vi "Add New Or Old Parameter.vi"(8 "old port?":bool, 9 "refresh listbox":T4[](array[typedef]), 10 "channel parameter":T1={"name"="", "default value"=0.0, "unit"="", "Parameter"={"start index"=0, "size"=1, "encoding"=enum."BNR", "signed"=FALSE, "scale multiplier"=1.0, "scale offset"=0.0}}) -> (1 "refresh listbox out":T4[](array[typedef]))   [LabVIEW 2020, in "AIM ARINC 429 System Explorer.lvlib" / "Implementation.lvlib"]
uses:
  Implementation.lvlib
  Types/Refresh Listbox.ctl
  Types/Refresh Symbols.ctl
  Shared/VS Channel Definition for Parameter.ctl
  Shared/Parameter Definition.ctl
  <vilib>/NI/NI VeriStand Encoding and Decoding/Encoding.ctl
  Refresh Constants.vi
  <vilib>/NI/NI VeriStand Encoding and Decoding/Encoding and Decoding.lvlib
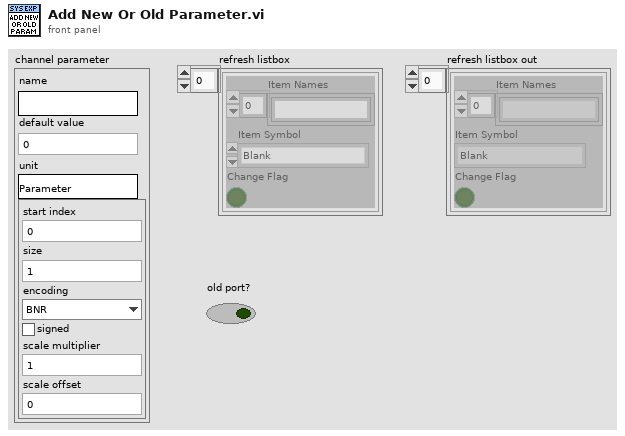
[diagram p1: front panel]
types:
  T1 = typedef "VS Channel Definition for Parameter.ctl" = cluster{"name":string, "default value":dbl, "unit":string, "Parameter":T2}
  T2 = typedef "Parameter Definition.ctl" = cluster{"start index":i32, "size":i32, "encoding":T3, "signed":bool, "scale multiplier":dbl, "scale offset":dbl}
  T3 = typedef "Encoding and Decoding.lvlib/Encoding.ctl" = enum16{"BNR", "BCD", "Discrete"}
  T4 = typedef "AIM ARINC 429 System Explorer.lvlib/Implementation.lvlib/Refresh Listbox.ctl" = cluster{"Item Names":string[], "Item Symbol":T5, "Change Flag":bool}
  T5 = typedef "AIM ARINC 429 System Explorer.lvlib/Implementation.lvlib/Refresh Symbols.ctl" = enum16{"Blank", "Port", "Incoming", "Outgoing", "Label", "Word", "Parameter", "ARINC-429", "Config Files", "Channel Spec", "Item"}
  T6 = typedef "AIM ARINC 429 System Explorer.lvlib/Implementation.lvlib/Parameter Strings.ctl" = cluster{"name":string, "default value":string, "unit":string, "start index":string, "size":string, "encoding":string, "signed":string, "scale multiplier":string, "scale offset":string}
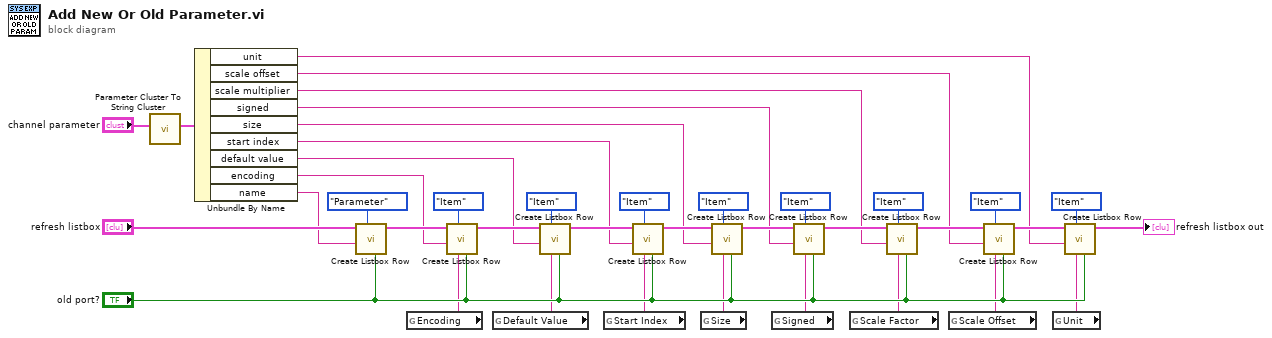
[diagram p0: block diagram]
diagram:
  n1 = call "Parameter Cluster To String Cluster.vi"("parameter"="channel parameter") -> ("parameter strings"=w18:T6)  [unwired: 10 in]
  n2 = Unbundle By Name(w18) -> ("unit"=w16:string, "scale offset"=w9:string, "scale multiplier"=w10:string, "signed"=w11:string, "size"=w12:string, "start index"=w13:string, "default value"=w14:string, "encoding"=w15:string, "name"=w17:string)
  n3 = call "Create Listbox Row.vi"("swap new and old (F)"="old port?", "refresh symbol (Blank)"=Refresh_Symbols."Parameter" ("Refresh Symbol (Blank)"), "new item"=w17, "refresh listbox"="refresh listbox") -> ("refresh listbox out"=w34:T4[])  [unwired: 7 in]
  n4 = global read "Refresh Constants.vi" "Encoding"() -> (w8:string)
  n5 = call "Create Listbox Row.vi"("swap new and old (F)"="old port?", "override name"=w8, "refresh symbol (Blank)"=Refresh_Symbols."Item" ("Refresh Symbol (Blank)"), "new item"=w15, "refresh listbox"=w34) -> ("refresh listbox out"=w32:T4[])  [unwired: 6 in]
  n6 = global read "Refresh Constants.vi" "Default Value"() -> (w7:string)
  n7 = call "Create Listbox Row.vi"("swap new and old (F)"="old port?", "override name"=w7, "refresh symbol (Blank)"=Refresh_Symbols."Item" ("Refresh Symbol (Blank)"), "new item"=w14, "refresh listbox"=w32) -> ("refresh listbox out"=w30:T4[])  [unwired: 6 in]
  n8 = global read "Refresh Constants.vi" "Start Index"() -> (w6:string)
  n9 = call "Create Listbox Row.vi"("swap new and old (F)"="old port?", "override name"=w6, "refresh symbol (Blank)"=Refresh_Symbols."Item" ("Refresh Symbol (Blank)"), "new item"=w13, "refresh listbox"=w30) -> ("refresh listbox out"=w28:T4[])  [unwired: 6 in]
  n10 = global read "Refresh Constants.vi" "Size"() -> (w5:string)
  n11 = call "Create Listbox Row.vi"("swap new and old (F)"="old port?", "override name"=w5, "refresh symbol (Blank)"=Refresh_Symbols."Item" ("Refresh Symbol (Blank)"), "new item"=w12, "refresh listbox"=w28) -> ("refresh listbox out"=w26:T4[])  [unwired: 6 in]
  n12 = global read "Refresh Constants.vi" "Signed"() -> (w4:string)
  n13 = call "Create Listbox Row.vi"("swap new and old (F)"="old port?", "override name"=w4, "refresh symbol (Blank)"=Refresh_Symbols."Item" ("Refresh Symbol (Blank)"), "new item"=w11, "refresh listbox"=w26) -> ("refresh listbox out"=w24:T4[])  [unwired: 6 in]
  n14 = global read "Refresh Constants.vi" "Scale Factor"() -> (w1:string)
  n15 = call "Create Listbox Row.vi"("swap new and old (F)"="old port?", "override name"=w1, "refresh symbol (Blank)"=Refresh_Symbols."Item" ("Refresh Symbol (Blank)"), "new item"=w10, "refresh listbox"=w24) -> ("refresh listbox out"=w22:T4[])  [unwired: 6 in]
  n16 = global read "Refresh Constants.vi" "Scale Offset"() -> (w2:string)
  n17 = call "Create Listbox Row.vi"("swap new and old (F)"="old port?", "override name"=w2, "refresh symbol (Blank)"=Refresh_Symbols."Item" ("Refresh Symbol (Blank)"), "new item"=w9, "refresh listbox"=w22) -> ("refresh listbox out"=w20:T4[])  [unwired: 6 in]
  n18 = global read "Refresh Constants.vi" "Unit"() -> (w3:string)
  n19 = call "Create Listbox Row.vi"("swap new and old (F)"="old port?", "override name"=w3, "refresh symbol (Blank)"=Refresh_Symbols."Item" ("Refresh Symbol (Blank)"), "new item"=w16, "refresh listbox"=w20) -> ("refresh listbox out"=→"refresh listbox out":T4[])  [unwired: 6 in]
